vi "UI - Read IO Variables.vi"(8 "error in (no error)":errorcluster, 11 "IO References":T1) -> (0 "error out":errorcluster, 1 "Temperature Values":dbl[](array[numeric]), 2 "Control Output Values":dbl[](array[numeric]), 3 "Control Input Values":dbl[](array[numeric]), 4 "Threshold Exceeded?":bool)   [LabVIEW 2017]
uses:
  controls/IO References.ctl
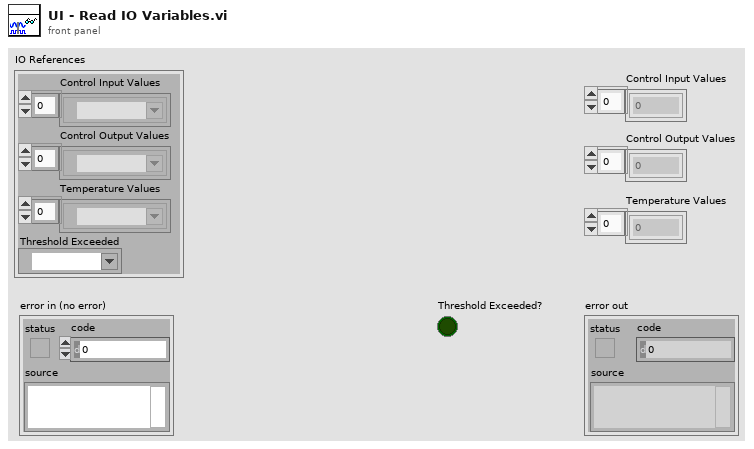
[diagram p1: front panel]
types:
  T1 = typedef "IO References.ctl" = cluster{"Control Input Values":refnum<k21>[], "Control Output Values":refnum<k21>[], "Temperature Values":refnum<k21>[], "Threshold Exceeded":refnum<k21>}
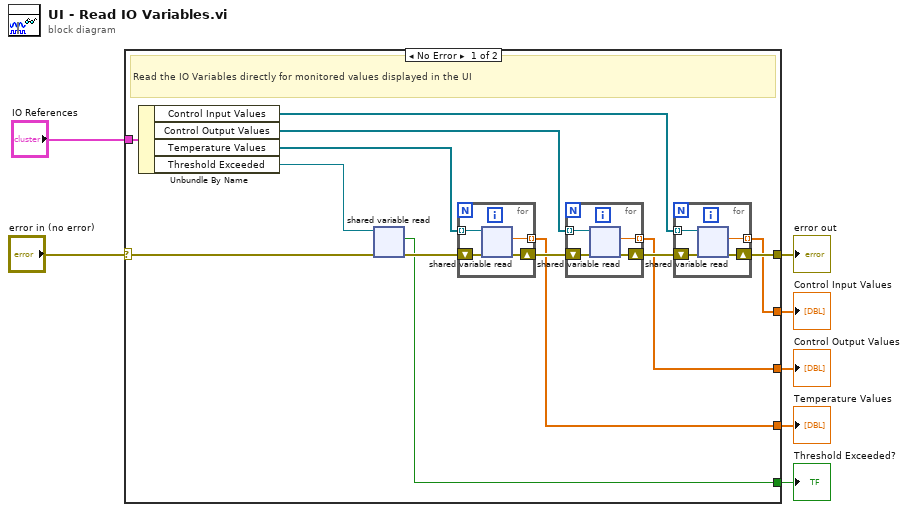
[diagram p0: block diagram]
diagram:
  n1 = case shown="No Error" "error in (no error)" {
    selector: "error in (no error)" -> [w8 w34]
    tunnel: "IO References" -> [w21 _]
    tunnel: [w13 w34] -> w6
    tunnel: [w12 _] -> w5
    tunnel: [w11 _] -> w4
    tunnel: [w10 _] -> w3
    tunnel: [w9 _] -> w2
    frame No Error {
      # "Read the IO Variables directly for monitored values displayed in the UI"
      n2 = Unbundle By Name(w21) -> ("Control Input Values"=w14:refnum<k21>[], "Control Output Values"=w16:refnum<k21>[], "Temperature Values"=w18:refnum<k21>[], "Threshold Exceeded"=w20:refnum<k21>)
      n3 = shared-variable-read(w20, w8) -> (w19:errorcluster, w12:bool)  [unwired: 2 out]
      n4 = for {
        shift-right: [w31] -> w17
        shift-left: w19 -> [w32]
        tunnel: w18 -> [w33] mode=indexing
        tunnel: [w30] -> w11 mode=indexing
        n5 = shared-variable-read(w33, w32) -> (w31:errorcluster, w30:dbl)  [unwired: 2 out]
      }
      n6 = for {
        shift-right: [w27] -> w15
        shift-left: w17 -> [w28]
        tunnel: w16 -> [w29] mode=indexing
        tunnel: [w26] -> w10 mode=indexing
        n7 = shared-variable-read(w29, w28) -> (w27:errorcluster, w26:dbl)  [unwired: 2 out]
      }
      n8 = for {
        shift-right: [w23] -> w13
        shift-left: w15 -> [w24]
        tunnel: w14 -> [w25] mode=indexing
        tunnel: [w22] -> w9 mode=indexing
        n9 = shared-variable-read(w25, w24) -> (w23:errorcluster, w22:dbl)  [unwired: 2 out]
      }
    }
    frame Error {
      # "Error"
    }
  }
  "error out" <- w6
  "Control Input Values" <- w2
  "Control Output Values" <- w3
  "Temperature Values" <- w4
  "Threshold Exceeded?" <- w5
